vi "Read Data.vi"(8 "error in (no error)":errorcluster, 11 "Abstruct Data Type in":refnum<class "Abstruct Data Type.lvclass">) -> (0 "error out":errorcluster, 2 "data":waveform(dbl)[](array[waveform]), 3 "Abstruct Data Type out":refnum<class "Abstruct Data Type.lvclass">)   [LabVIEW 2020, in "Abstruct Data Type.lvclass"]
uses:
  Abstruct Data Type.lvclass
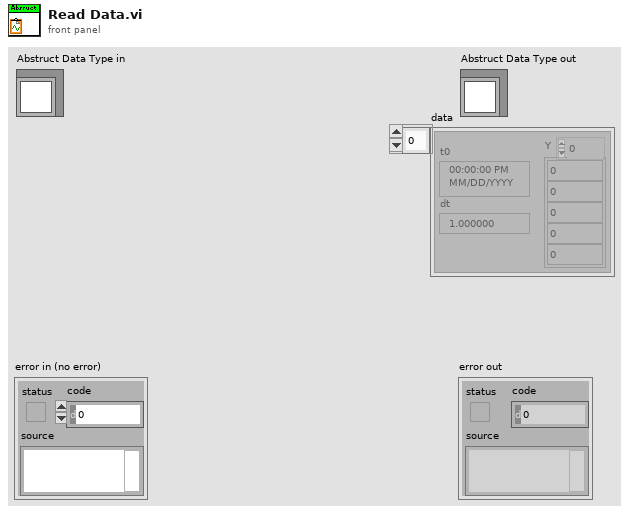
[diagram p1: front panel]
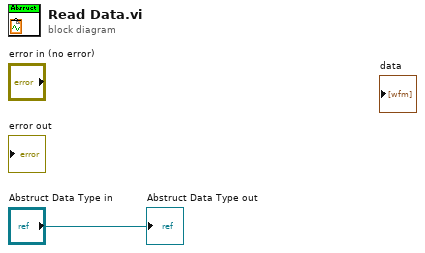
[diagram p0: block diagram]
diagram:
  "Abstruct Data Type out" <- "Abstruct Data Type in"
